vi "Update Device Measurement.vi"(8 "error in":errorcluster, 11 "Manual Control in":refnum<class "Manual Control.lvclass">) -> (0 "error out":errorcluster, 3 "Manual Control out":refnum<class "Manual Control.lvclass">)   [LabVIEW 2018, in "Manual Control Actor.lvlib" / "Manual Control.lvclass"]
uses:
  Manual Control.lvclass
  C:/Users/Administrator/Desktop/2018LabVIEW EMS/EMS Generic Actor/EMS Generic/EMS Generic.lvclass
  C:/Program Files (x86)/National Instruments/LabVIEW 2018/vi.lib/ActorFramework/Actor/Actor.lvclass
  Manual Control.lvclass/Manual Control.ctl
  <vilib>/ORNL/CSEISMIC DDS/CSEISMIC DDS Base/Data Types/DER_Measurement.ctl
  <vilib>/ORNL/CSEISMIC DDS/CSEISMIC DDS Base/Data Types/Controls/DeviceID.ctl
  <vilib>/ActorFramework/Actor/Actor.lvclass/Actor.ctl
  EMS Generic Actor/EMS Generic/EMS Generic.lvclass/EMS Generic.ctl
  EMS Generic Actor/EMS Generic Messages/Return DER_Measurement Msg/Return DER_Measurement Msg.lvclass/Return DER_Measurement Msg.ctl
  <vilib>/ActorFramework/Message Enqueuer/Message Enqueuer.lvclass/Message Enqueuer.ctl
  <vilib>/ActorFramework/Message Enqueuer/Enqueue.vi
  EMS Generic Actor/EMS Generic Messages/Return DER_Measurement Msg/Return DER_Measurement Msg.lvclass
  C:/Program Files (x86)/National Instruments/LabVIEW 2018/vi.lib/ActorFramework/Message/Message.lvclass
  <vilib>/ActorFramework/Message Priority Queue/Priority Enqueue.vi
  EMS Generic Actor/EMS Generic/EMS Generic.lvclass
  <vilib>/ActorFramework/Actor/Actor.lvclass
  <vilib>/ORNL/CSEISMIC DDS/CSEISMIC DDS Base/CSEISMIC DDS.lvclass
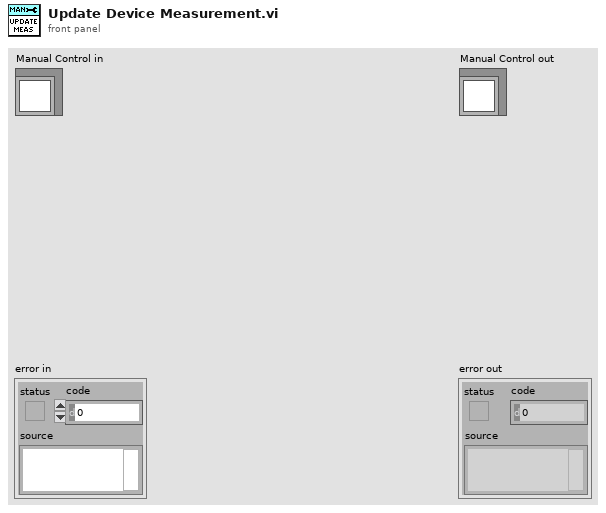
[diagram p1: front panel]
types:
  T1 = typedef "CSEISMIC DDS.lvlib/CSEISMIC DDS.lvclass/DER_Measurement.ctl" = cluster{"DeviceID":T2, "Voltage":dbl[], "Current":dbl[], "RealPower":dbl[], "ReactivePower":dbl[], "LineConfig":u8[], "Frequency":dbl}
  T2 = typedef "CSEISMIC DDS.lvlib/CSEISMIC DDS.lvclass/DeviceID.ctl" = string
  T3 = typedef "CSEISMIC DDS.lvlib/CSEISMIC DDS.lvclass/SmartRelay_Measurement.ctl" = cluster{"DeviceID":T2, "PrimaryVoltage":dbl[], "SecondaryVoltage":dbl[], "Current":dbl[], "RealPower":dbl[], "ReactivePower":dbl[], "LineConfig":u8[], "Frequency":dbl}
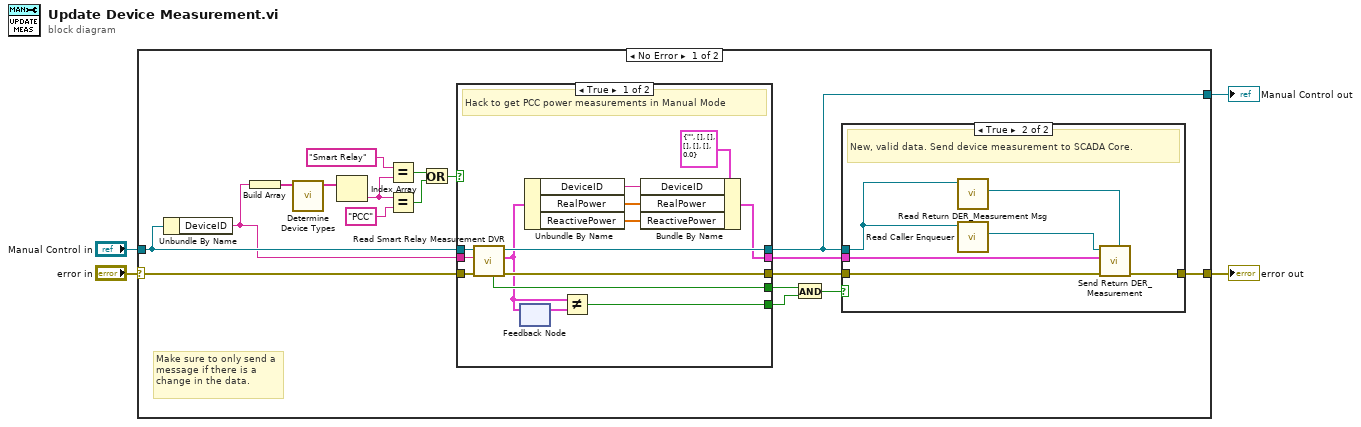
[diagram p0: block diagram]
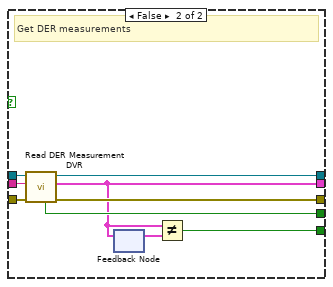
[diagram p2: hidden frame]
diagram:
  n1 = case shown="No Error" "error in" {
    selector: "error in" -> [w14 w54]
    tunnel: [w20 w54] -> w3
    tunnel: [w22 w53] -> w1
    tunnel: "Manual Control in" -> [w15 w53]
    frame No Error {
      # "Make sure to only send a message if there is a change in the data."
      n2 = Unbundle By Name(w15) -> ("DeviceID"=w13:T2)
      n3 = Build Array(w13) -> (w12:T2[])
      n4 = call "Determine Device Types.vi"("DeviceIDs"=w12) -> ("Device Classes"=w11:string[])  [unwired: 9 in]
      n5 = Index Array(array=w11) -> (element=w9:string)  [unwired: 1 in]
      n6 = Equal?(x="Smart Relay", y=w9) -> (x = y?=w7:bool)
      n7 = Equal?(x=w9, y="PCC") -> (x = y?=w6:bool)
      n8 = Or(x=w7, y=w6) -> (x .or. y?=w5:bool)
      n9 = case shown="True" w5 {
        tunnel: w15 -> [w36 w45]
        tunnel: w13 -> [w35 w44]
        tunnel: w14 -> [w34 w43]
        tunnel: [w33 w42] -> w22
        tunnel: [w32 w41] -> w21
        tunnel: [w31 w40] -> w19
        tunnel: [w23 w39] -> w17
        tunnel: [w29 w37] -> w16
        frame True {
          # "Hack to get PCC power measurements in Manual Mode"
          n10 = call "Read Smart Relay Measurement DVR.vi"("error in"=w34, "DeviceID"=w35, "EMS Generic in"=w36) -> ("error out"=w32:errorcluster, "SmartRelay_Measurement"=w28:T3, "EMS Generic out"=w33:refnum<class "Manual Control.lvclass">, "valid?"=w31:bool)  [unwired: 5 in]
          n11 = feedback #1() -> (w30:T3)  [unwired: 1 in]
          n12 = feedback-in #1(w28) -> ()
          n13 = Unbundle By Name(w28) -> ("DeviceID"=w26:T2, "RealPower"=w25:dbl[], "ReactivePower"=w24:dbl[])
          n14 = Not Equal?(x=w28, y=w30) -> (x != y?=w29:bool)
          n15 = Bundle By Name(cluster=T1 {"DeviceID"="", "Voltage"=[], "Current"=[], "RealPower"=[], "ReactivePower"=[], "LineConfig"=[], "Frequency"=0.0} ("DER_Measurement"), "DeviceID"=w26, "RealPower"=w25, "ReactivePower"=w24) -> (w23:T1)
        }
        frame False {
          # "Get DER measurements"
          n16 = call "Read DER Measurement DVR.vi"("error in"=w43, "DeviceID"=w44, "EMS Generic in"=w45) -> ("error out"=w41:errorcluster, "DER_Measurement"=w39:T1, "EMS Generic out"=w42:refnum<class "Manual Control.lvclass">, "valid?"=w40:bool)  [unwired: 5 in]
          n17 = feedback #2() -> (w38:T1)  [unwired: 1 in]
          n18 = feedback-in #2(w39) -> ()
          n19 = Not Equal?(x=w39, y=w38) -> (x != y?=w37:bool)
        }
      }
      n20 = And(x=w19, y=w16) -> (x .and. y?=w18:bool)
      n21 = case shown="True" w18 {
        tunnel: w22 -> [_ w52]
        tunnel: w17 -> [_ w48]
        tunnel: w21 -> [w46 w51]
        tunnel: [w46 w50] -> w20
        frame False {
          # "#TODO Should update status on Master Controller Core"
          # "No measurement data available for specified device"
        }
        frame True {
          # "New, valid data. Send device measurement to SCADA Core."
          n22 = call "Read Return DER_Measurement Msg.vi"("EMS Generic in"=w52) -> ("Return DER_Measurement Msg"=w47:refnum<class "Return DER_Measurement Msg.lvclass">)  [unwired: 9 in, 1 out]
          n23 = call <vilib>:"Read Caller Enqueuer.vi"("Actor"=w52) -> ("Caller Enqueuer"=w49:refnum<class "Message Enqueuer.lvclass">)  [unwired: 10 in]
          n24 = call "Send Return DER_Measurement.vi"("Message Type"=w47, "error in (no error)"=w51, "DER_Measurement"=w48, "Message Enqueuer"=w49) -> ("error out"=w50:errorcluster)  [unwired: 6 in, 1 out]
        }
      }
    }
    frame Error {
    }
  }
  "error out" <- w3
  "Manual Control out" <- w1
